vi "SRDG535.PC Set Delay.vi"(0 "i ref in":refnum<vi>, 2 "Delay Settings":T1 {"CH D"."Delay (s)" format="%#_13g"; "CH D"."rel to" scale=0.0..3.0; "CH C"."Delay (s)" format="%#_13g"; "CH C"."rel to" scale=0.0..3.0; "CH B"."Delay (s)" format="%#_13g"; "CH B"."rel to" scale=0.0..3.0; "CH A"."Delay (s)" format="%#_13g"; "CH A"."rel to" scale=0.0..3.0}, 5 "error IO":errorcluster) -> (14 "i ref out":refnum<vi>, 19 "error out":errorcluster)   [LabVIEW 2014, in "SRDG535.lvlib"]
doc: "This VI communicates with the hardware, sets own attributes and GUI elements."
uses:
  SRDG535.lvlib
  SRDG535.Delay.ctl
  non_GPL/instr.lib/srdg535/Stanford Research DG535 - Driver np.lvlib
  CSPhelix/PH_Common/PH_Common.lvlib
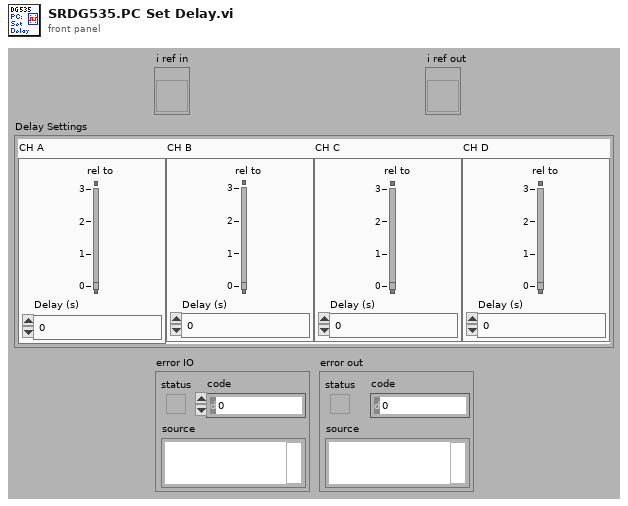
[diagram p1: front panel]
types:
  T1 = typedef "SRDG535.lvlib/SRDG535.Delay.ctl" = cluster{"CH A":cluster{"rel to":u32, "Delay (s)":dbl}, "CH B":cluster{"rel to":u32, "Delay (s)":dbl}, "CH C":cluster{"rel to":u32, "Delay (s)":dbl}, "CH D":cluster{"rel to":u32, "Delay (s)":dbl}}
  T2 = typedef "SRDG535.lvlib/SRDG535.i attribute.ctl" = cluster{"GPIB address":string, "Device error":errorcluster, "GUI Refs":cluster{"Delete":refnum<vi>, "Device Error":refnum<vi>, "Information":refnum<vi>, "Output":refnum<vi>, "Delay":refnum<vi>, "Trigger":refnum<vi>}, "Output Settings":T3, "Service ID Rate":i32, "Service IDs Channelinfo":i32[], "Delay Settings":T1, "Trigger Settings":T5}
  T3 = typedef "SRDG535.lvlib/SRDG535.Output.ctl" = cluster{"CH T0":T4, "CH A":T4, "CH B":T4, "CH AB":T4, "CH C":T4, "CH D":T4, "CH CD":T4}
  T4 = typedef "SRDG535.lvlib/SRDG535.Channel Output.ctl" = cluster{"Inversion":bool, "Amplitude (V)":dbl, "Offset (V)":dbl, "Mode":i32, "Load":bool}
  T5 = typedef "SRDG535.lvlib/SRDG535.Trigger.ctl" = cluster{"trigger":u32, "Impedance":bool, "Slope":bool, "burst count":i32, "external level (V)":sgl, "Internal/Burst Rate (Hz)":dbl, "Burst Period":i32}
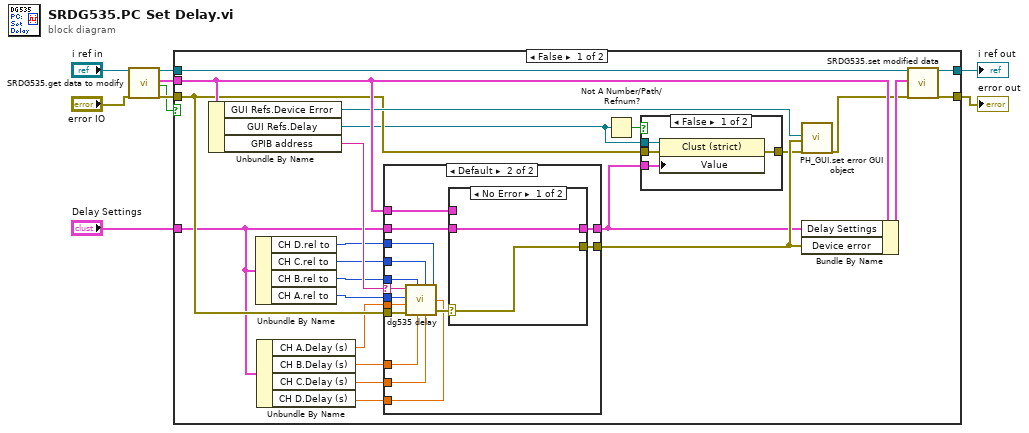
[diagram p0: block diagram]
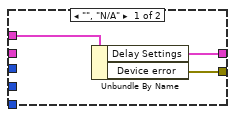
[diagram p3: hidden frame]
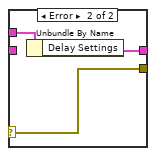
[diagram p4: hidden frame]
diagram:
  n1 = call "SRDG535.get data to modify.vi"("i ref in"="i ref in", "error in (no error)"="error IO") -> ("i ref out"=w5:refnum<vi>, "i attribute"=w9:T2, "timed out"=w2:bool, "error out"=w7:errorcluster)  [unwired: 14 in]
  n2 = case shown="False" w2 {
    tunnel: w9 -> [w32 _]
    tunnel: [w30 w61] -> w8
    tunnel: w7 -> [w23 w61]
    tunnel: [w29 w62] -> w6
    tunnel: w5 -> [w28 w62]
    tunnel: "Delay Settings" -> [w14 _]
    frame False {
      n3 = Unbundle By Name(w32) -> ("GUI Refs.Device Error"=w25:refnum<vi>, "GUI Refs.Delay"=w21:refnum<vi>, "GPIB address"=w20:string)
      n4 = Unbundle By Name(w14) -> ("CH D.rel to"=w10:u32, "CH C.rel to"=w11:u32, "CH B.rel to"=w12:u32, "CH A.rel to"=w13:u32)
      n5 = Unbundle By Name(w14) -> ("CH A.Delay (s)"=w18:dbl, "CH B.Delay (s)"=w17:dbl, "CH C.Delay (s)"=w16:dbl, "CH D.Delay (s)"=w15:dbl)
      n6 = case shown="Default" w20 {
        selector: w20 -> [_ w55]
        tunnel: w23 -> [_ w54]
        tunnel: [w39 w51] -> w26
        tunnel: w32 -> [w40 w52]
        tunnel: [w38 w49] -> w19
        tunnel: w14 -> [_ w50]
        tunnel: w18 -> [_ w48]
        tunnel: w17 -> [_ w47]
        tunnel: w16 -> [_ w46]
        tunnel: w15 -> [_ w45]
        tunnel: w13 -> [_ w44]
        tunnel: w12 -> [_ w43]
        tunnel: w11 -> [_ w42]
        tunnel: w10 -> [_ w41]
        frame "", "N/A" {
          n7 = Unbundle By Name(w40) -> ("Delay Settings"=w38:T1, "Device error"=w39:errorcluster)
        }
        frame Default {
          n8 = call "dg535 delay.vi"("C"=w46, "D"=w45, "D="=w41, "C="=w42, "B"=w47, "error in"=w54, "A"=w48, "B="=w43, "A="=w44, "GPIB address"=w55) -> ("error out"=w53:errorcluster)
          n9 = case shown="No Error" w53 {
            selector: w53 -> [w57 w58]
            tunnel: w52 -> [_ w60]
            tunnel: [w57 w58] -> w51
            tunnel: w50 -> [w56 _]
            tunnel: [w56 w59] -> w49
            frame No Error {
            }
            frame Error {
              n10 = Unbundle By Name(w60) -> ("Delay Settings"=w59:T1)
            }
          }
        }
      }
      n11 = Not A Number/Path/Refnum?(number/path/refnum=w21) -> (NaN/Path/Refnum?=w22:bool)
      n12 = case shown="False" w22 {
        tunnel: [w36 w37] -> w24
        tunnel: w23 -> [w35 w37]
        tunnel: w21 -> [w34 _]
        tunnel: w19 -> [w33 _]
        frame False {
          n13 = property class="Clust (strict)"(reference=w34, error in=w35, "Value"=w33) -> (error out=w36:errorcluster)  [unwired: 1 out]
        }
        frame True {
        }
      }
      n14 = call "PH_GUI.set error GUI object.vi"("GUI Refs.Device Error"=w25, "error to set"=w26, "error in (no error)"=w24) -> ("error out"=w27:errorcluster)  [unwired: 16 in]
      n15 = Bundle By Name(cluster=w32, "Delay Settings"=w19, "Device error"=w26) -> (w31:T2)
      n16 = call "SRDG535.set modified data.vi"("i ref in"=w28, "i attribute"=w31, "error in (no error)"=w27) -> ("i ref out"=w29:refnum<vi>, "error out"=w30:errorcluster)  [unwired: 15 in]
    }
    frame True {
    }
  }
  "error out" <- w8
  "i ref out" <- w6
